vi "Memory.Array.Get Allocated Size.vi"(8 "error in (no error)":errorcluster, 11 "Array in":refnum<class "Memory.Array.Void.lvclass">) -> (0 "error out":errorcluster, 2 "allocated size":i64 format="%d bytes", 3 "Array out":refnum<class "Memory.Array.Void.lvclass">)   [LabVIEW 2016, in "Memory Manager.lvlib" / "Memory.Array.Void.lvclass"]
uses:
  Memory.Array.Void.lvclass
  Memory.Array.Void.lvclass/Memory.Array.Void.ctl
  Pointer/Pointer.Void/Memory.Pointer.Void.lvclass/Memory.Pointer.Void.ctl
  Pointer/Pointer.Void/Memory.Pointer.Void.lvclass
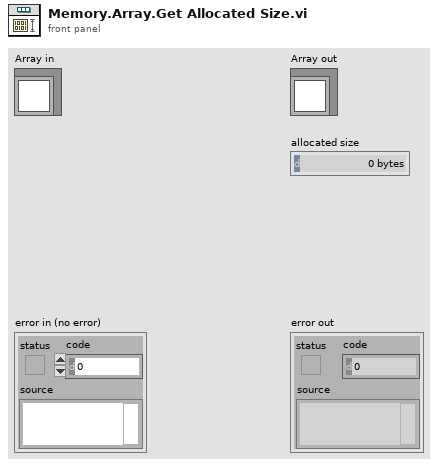
[diagram p1: front panel]
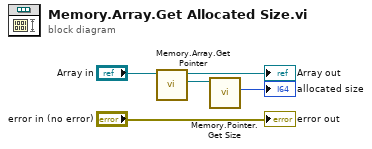
[diagram p0: block diagram]
diagram:
  n1 = call "Memory.Array.Get Pointer.vi"("Array in"="Array in") -> ("Pointer"=w4:refnum<class "Memory.Pointer.Void.lvclass">, "Array out"=→"Array out":refnum<class "Memory.Array.Void.lvclass">)  [unwired: 8 in, 1 out]
  n2 = call "Memory.Pointer.Get Size.vi"("Pointer in"=w4) -> ("size"=→"allocated size":u64)  [unwired: 8 in, 2 out]
  "error out" <- "error in (no error)"
